vi "Write Unit ID.vi"(8 "error in":errorcluster, 10 "unit ID":u8, 11 "transmission data unit in":refnum<class "Transmission Data Unit.lvclass">) -> (0 "error out":errorcluster, 3 "transmission data unit out":refnum<class "Transmission Data Unit.lvclass">)   [LabVIEW 2013, in "Modbus Library - Advance.lvlib" / "Transmission Data Unit.lvclass"]
doc: "Sets the unit ID of the device."
uses:
  Transmission Data Unit.lvclass
  Transmission Data Unit.lvclass/Transmission Data Unit.ctl
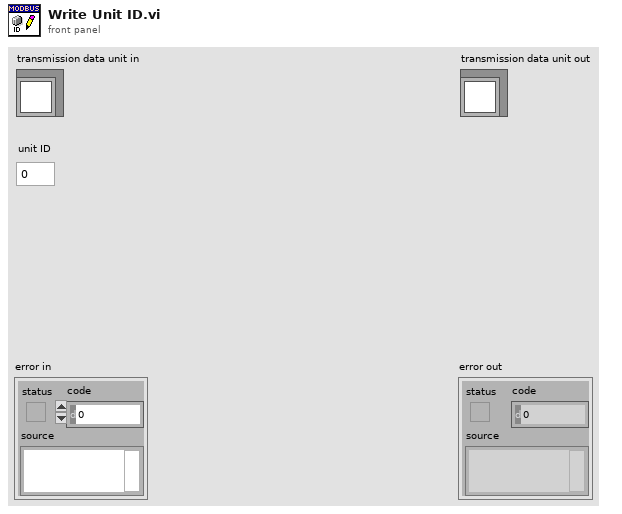
[diagram p1: front panel]
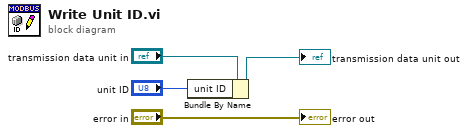
[diagram p0: block diagram]
diagram:
  n1 = Bundle By Name(cluster="transmission data unit in", "unit ID"="unit ID") -> (→"transmission data unit out":refnum<class "Transmission Data Unit.lvclass">)
  "error out" <- "error in"
